vi "GUI.ConfigureUI.vi"(8 "error in (no error)":errorcluster) -> (0 "error out":errorcluster, 1 "Log Path out":path, 2 "Canceled?":bool, 3 "gRPC Info":T4)   [LabVIEW 2026, in "XNET Bus Monitor Client.lvlib"]
uses:
  XNET Bus Monitor Client.lvlib
  Types/gRPC.ConnectionInfo.ctl
  <vilib>/gRPC/LabVIEW gRPC Library/Shared/grpcId.ctl
  bus_monitor_client/RPC Messages/ni_bus_monitor_api_Session.ctl
  bus_monitor_client/RPC Messages/ni_bus_monitor_api_CanMode.ctl
  bus_monitor_client/RPC Messages/ni_bus_monitor_api_FdIsoMode.ctl
  bus_monitor_client/RPC Messages/ni_bus_monitor_api_Termination.ctl
  bus_monitor_client/RPC Messages/ni_bus_monitor_api_InitializeSettingsRequest.ctl
  bus_monitor_client/RPC Messages/ni_bus_monitor_api_ConnectSettings.ctl
  bus_monitor_client/bus_monitor_client.lvlib
  <vilib>/gRPC/LabVIEW gRPC Library/grpc-lvsupport-release.lvlib
panel:
  in  "Log Folder Path":path
  in  "FD Baud_Rate":u64 format="%.0x"
  in  "Baud Rate":u64
  in  "Termination":T1
  in  "FD ISO Mode":T2
  in  "CAN Mode":T3
  in  "Cancel":bool
  in  "Connect":bool
  out "Found Port":u64
  in  "Check Connection":bool
  in  "Service Name":string
  in  "IP Address":string
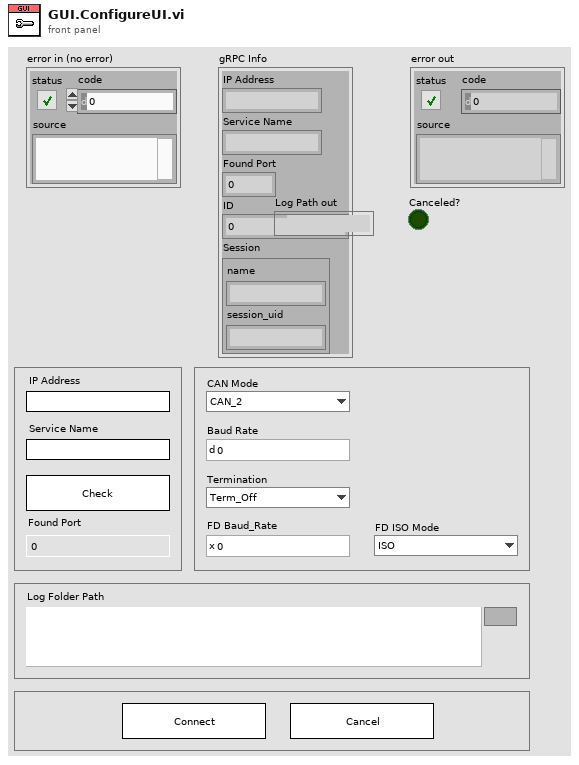
[diagram p1: front panel]
types:
  T1 = typedef "bus_monitor_client.lvlib/ni_bus_monitor_api_Termination.ctl" = enum32{"Term_Off", "Term_On"}
  T2 = typedef "bus_monitor_client.lvlib/ni_bus_monitor_api_FdIsoMode.ctl" = enum32{"ISO", "Non_ISO", "ISO_Legacy"}
  T3 = typedef "bus_monitor_client.lvlib/ni_bus_monitor_api_CanMode.ctl" = enum32{"CAN_2", "CAN_FD", "CAN_FD_BRS"}
  T4 = typedef "XNET Bus Monitor Client.lvlib/gRPC.ConnectionInfo.ctl" = cluster{"IP Address":string, "Service Name":string, "Found Port":u64, "ID":T5, "Session":T6}
  T5 = typedef "grpc-lvsupport-release.lvlib/grpcId.ctl" = u64
  T6 = typedef "bus_monitor_client.lvlib/ni_bus_monitor_api_Session.ctl" = cluster{"name":string, "session_uid":string}
  T7 = enum8{"Enabled", "Disabled", "Disabled and Grayed Out"}
  T8 = typedef "bus_monitor_client.lvlib/ni_bus_monitor_api_InitializeSettingsRequest.ctl" = cluster{"name":string, "connect_settings":T9, "default_filter_ids":u32[]}
  T9 = typedef "bus_monitor_client.lvlib/ni_bus_monitor_api_ConnectSettings.ctl" = cluster{"port":string, "can_mode":T3, "termination":T1, "baud_rate":u64, "fd_baud_rate":u64, "fd_iso_mode":T2}
  T10 = typedef "bus_monitor_client.lvlib/ni_bus_monitor_api_InitializeSettingsReply.ctl" = cluster{"session":T6, "error":T11}
  T11 = typedef "bus_monitor_client.lvlib/ni_bus_monitor_api_ErrorInfo.ctl" = errorcluster
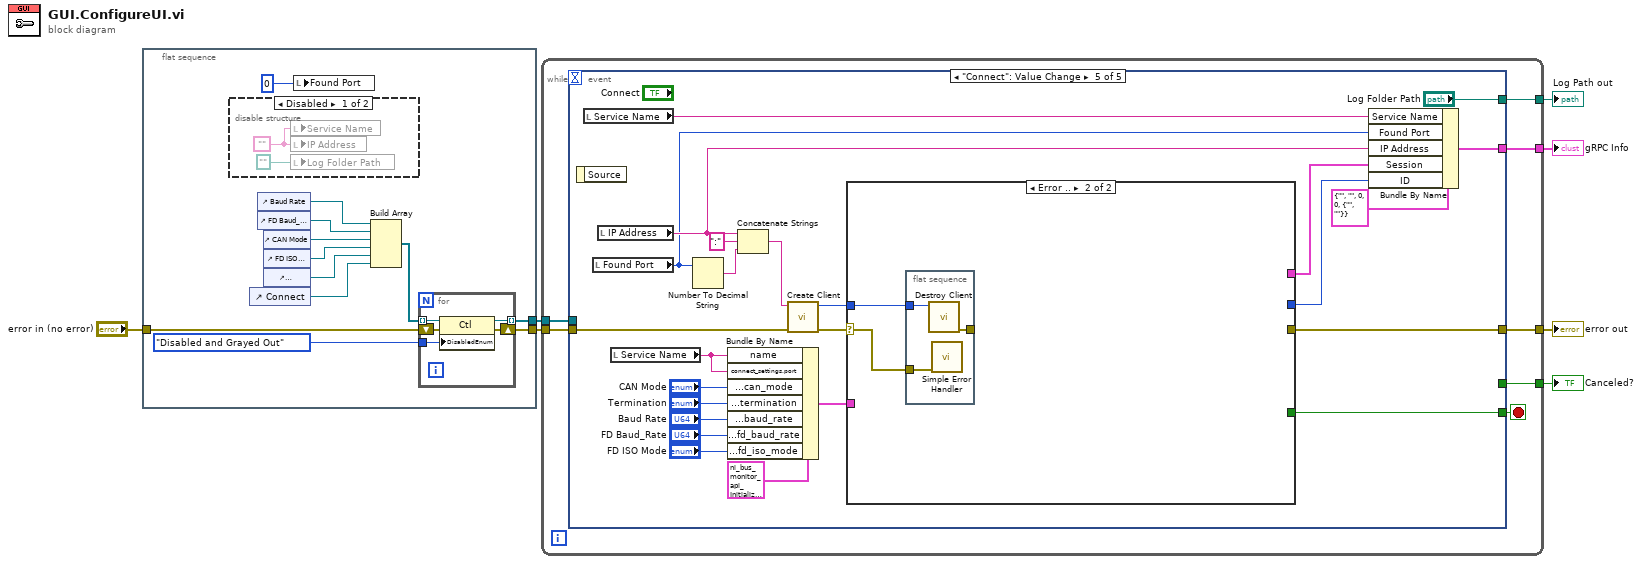
[diagram p0: block diagram]
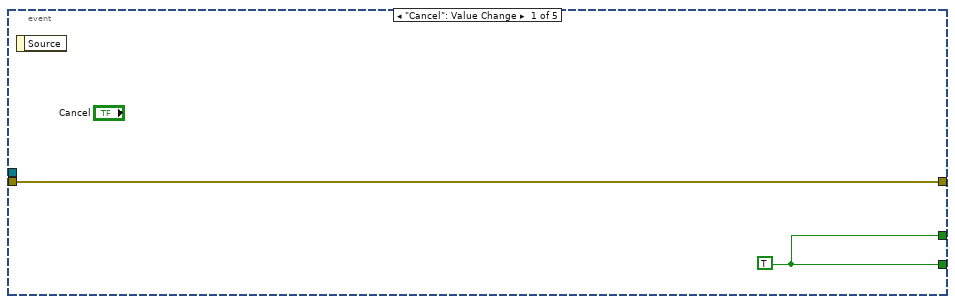
[diagram p3: hidden frame]
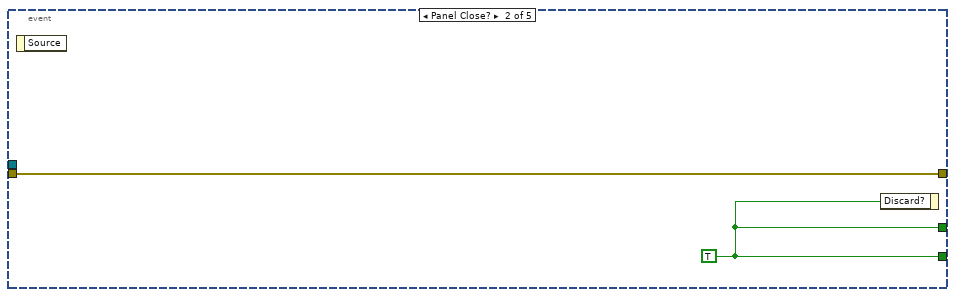
[diagram p4: hidden frame]
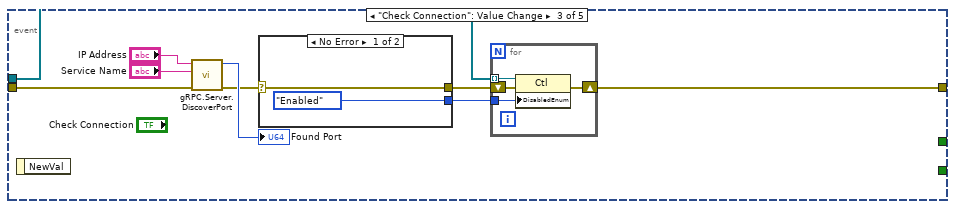
[diagram p5: hidden frame]
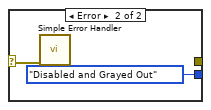
[diagram p6: hidden frame]
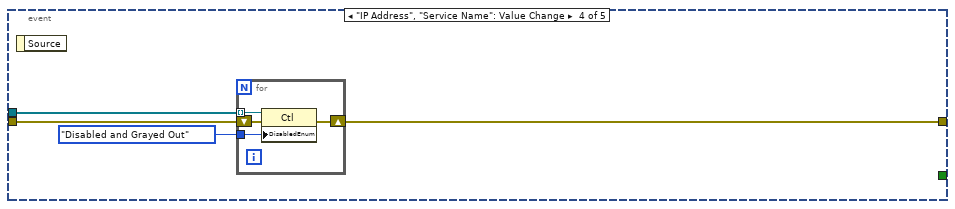
[diagram p7: hidden frame]
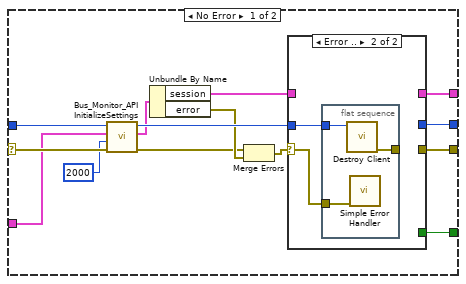
[diagram p8: hidden frame]
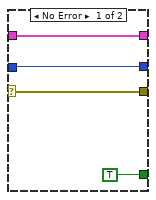
[diagram p9: hidden frame]
diagram:
  n1 = flat-sequence {
    tunnel: [w18] -> w6
    tunnel: [w17] -> w5
    tunnel: "error in (no error)" -> [w15]
    frame #0 {
      n2 = disable-structure shown="Disabled" {
        frame Disabled {
          w21 = ""
          n3 = local write "Service Name"(w21) -> ()
          n4 = local write "IP Address"(w21) -> ()
          n5 = local write "Log Folder Path"(path "") -> ()
        }
        frame Enabled {
        }
      }
      n6 = control-ref of="Connect"() -> (w9:refnum<vi>)
      n7 = control-ref of="Baud Rate"() -> (w14:refnum<vi>)
      n8 = control-ref of="FD Baud_Rate"() -> (w13:refnum<vi>)
      n9 = control-ref of="CAN Mode"() -> (w12:refnum<vi>)
      n10 = control-ref of="FD ISO Mode"() -> (w11:refnum<vi>)
      n11 = control-ref of="Termination"() -> (w10:refnum<vi>)
      n12 = local write "Found Port"(u64 0 ("Found Port")) -> ()
      n13 = Build Array(w14, w13, w12, w11, w10, w9) -> (w8:refnum<vi>[])
      n14 = for {
        tunnel: T7."Disabled and Grayed Out" ("Disabled") -> [w26]
        tunnel: [w25] -> w18 mode=indexing
        shift-right: [w24] -> w17
        shift-left: w15 -> [w23]
        tunnel: w8 -> [w22] mode=indexing
        n15 = property class="Ctl"(reference=w22, error in=w23, "DisabledEnum"=w26) -> (reference out=w25:refnum<vi>, error out=w24:errorcluster)
      }
    }
  }
  n16 = while {
    tunnel: [w32] -> w7
    tunnel: w6 -> [w31]
    tunnel: w5 -> [w30]
    tunnel: [w29] -> w3
    tunnel: [w28] -> w4
    tunnel: [w27] -> w1
    stop <- w33 stop-if-true
    n17 = event shown="[4] \"Connect\": Value Change" {
      selector: _ -> [_ _ _ _ _]
      dyn-events: _ -> [_ _ _ _ _]
      timeout: _ -> [_ _ _ _ _]
      tunnel: [w35 w37 _ _ w81] -> w33
      tunnel: [w35 w37 _ _ _] -> w32
      tunnel: w31 -> [_ _ w41 w57 _]
      tunnel: w30 -> [w34 w36 w44 w56 w83]
      tunnel: [w34 w36 w38 w55 w80] -> w29
      tunnel: [_ _ _ _ w78] -> w28
      tunnel: [_ _ _ _ "Log Folder Path"] -> w27
      event "Cancel": Value Change {
        w35 = TRUE
        n18 = event-data() -> ()  [unwired: 1 in, 1 out]
      }
      event Panel Close? {
        w37 = TRUE
        n19 = event-data() -> ()  [unwired: 1 in, 1 out]
        n20 = event-data("Discard?"=w37) -> ()  [unwired: 1 in, 1 out]
      }
      event "Check Connection": Value Change {
        n21 = event-data() -> ()  [unwired: 1 in, 1 out]
        n22 = call "gRPC.Server.DiscoverPort.vi"("error in (no error)"=w44, "Name"="Service Name", "IP Address"="IP Address") -> ("error out"=w42:errorcluster, "Port"=→"Found Port":i32)  [unwired: 7 in]
        n23 = case shown="No Error" w42 {
          selector: w42 -> [w52 w53]
          tunnel: [w52 _] -> w40
          tunnel: [T7."Enabled" ("Disabled") T7."Disabled and Grayed Out" ("Disabled")] -> w39
          frame No Error {
          }
          frame Error {
            n24 = call <vilib>:"Simple Error Handler.vi"("error in (no error)"=w53) -> ()  [unwired: 4 in, 5 out]
          }
        }
        n25 = for {
          tunnel: w41 -> [w50] mode=indexing
          tunnel: w39 -> [w48]
          shift-right: [w47] -> w38
          shift-left: w40 -> [w49]
          n26 = property class="Ctl"(reference=w50, error in=w49, "DisabledEnum"=w48) -> (error out=w47:errorcluster)  [unwired: 1 out]
        }
      }
      event "IP Address", "Service Name": Value Change {
        n27 = event-data() -> ()  [unwired: 1 in, 1 out]
        n28 = for {
          tunnel: T7."Disabled and Grayed Out" ("Disabled") -> [w62]
          tunnel: w57 -> [w61] mode=indexing
          shift-right: [w59] -> w55
          shift-left: w56 -> [w60]
          n29 = property class="Ctl"(reference=w61, error in=w60, "DisabledEnum"=w62) -> (error out=w59:errorcluster)  [unwired: 1 out]
        }
      }
      event "Connect": Value Change {
        n30 = event-data() -> ()  [unwired: 1 in, 1 out]
        n31 = local read "Service Name"() -> (w67:string)
        n32 = local read "Found Port"() -> (w76:u64)
        n33 = local read "IP Address"() -> (w79:string)
        n34 = local read "Service Name"() -> (w64:string)
        n35 = Number To Decimal String(number=w76) -> (decimal integer string=w85:string)  [unwired: 1 in]
        n36 = Bundle By Name(cluster=T8 {"name"="", "connect_settings"={"port"="", "can_mode"=enum."CAN_2", "termination"=enum."Term_Off", "baud_rate"=0, "fd_baud_rate"=0, "fd_iso_mode"=enum."ISO"}, "default_filter_ids"=[]} ("Request Data"), "name"=w64, "connect_settings.port"=w64, "connect_settings.can_mode"="CAN Mode", "connect_settings.termination"="Termination", "connect_settings.baud_rate"="Baud Rate", "connect_settings.fd_baud_rate"="FD Baud_Rate", "connect_settings.fd_iso_mode"="FD ISO Mode") -> (w68:T8)
        n37 = Concatenate Strings(w79, ":" ("string"), w85) -> (w84:string)
        n38 = call "Create Client.vi"("error in"=w83, "address"=w84) -> ("error out"=w82:errorcluster, "gRPC ID Out"=w75:T5)  [unwired: 8 in]
        n39 = case shown="Error .." w82 {
          selector: w82 -> [w99 w111]
          tunnel: [w100 _] -> w81
          tunnel: [w95 _] -> w80
          tunnel: w75 -> [w97 w110]
          tunnel: w68 -> [w90 _]
          tunnel: [w89 _] -> w66
          tunnel: [w87 _] -> w63
          frame No Error {
            n40 = call "Bus_Monitor_API InitializeSettings.vi"("error in"=w99, "timeout (ms)"=2000, "Request Data"=w90, "gRPC ID"=w97) -> ("error out"=w92:errorcluster, "Response Data"=w94:T10, "gRPC ID out"=w96:T5)  [unwired: 5 in]
            n41 = Unbundle By Name(w94) -> ("session"=w88:T6, "error"=w93:T11)
            n42 = Merge Errors(w92, w93) -> (w91:errorcluster)
            n43 = case shown="Error .." w91 {
              selector: w91 -> [w103 w106]
              tunnel: [TRUE _] -> w100
              tunnel: w96 -> [w102 w105]
              tunnel: [w103 _] -> w95
              tunnel: [w102 _] -> w89
              tunnel: w88 -> [w101 _]
              tunnel: [w101 _] -> w87
              frame No Error {
              }
              frame Error {
                n44 = flat-sequence {
                  tunnel: w106 -> [w109]
                  tunnel: w105 -> [w107]
                  tunnel: [w108] -> _
                  frame #0 {
                    n45 = call "Destroy Client.vi"("gRPC ID"=w107) -> ("error out"=w108:errorcluster)  [unwired: 10 in]
                    n46 = call <vilib>:"Simple Error Handler.vi"("error in (no error)"=w109) -> ()  [unwired: 4 in, 5 out]
                  }
                }
              }
            }
          }
          frame Error {
            n47 = flat-sequence {
              tunnel: w111 -> [w114]
              tunnel: w110 -> [w113]
              tunnel: [w112] -> _
              frame #0 {
                n48 = call "Destroy Client.vi"("gRPC ID"=w113) -> ("error out"=w112:errorcluster)  [unwired: 10 in]
                n49 = call <vilib>:"Simple Error Handler.vi"("error in (no error)"=w114) -> ()  [unwired: 4 in, 5 out]
              }
            }
          }
        }
        n50 = Bundle By Name(cluster=T4 {"IP Address"="", "Service Name"="", "Found Port"=0, "ID"=0, "Session"={"name"="", "session_uid"=""}}, "Service Name"=w67, "Found Port"=w76, "IP Address"=w79, "Session"=w63, "ID"=w66) -> (w78:T4)
      }
    }
  }
  "Canceled?" <- w7
  "gRPC Info" <- w4
  "error out" <- w3
  "Log Path out" <- w1
